vi "am_write_subvi.vi"(6 "Data to Write":u8 format="%.0x", 8 "error in (no error)":errorcluster, 9 "Memory ADD":u16=80 max=1023 format="%.0x", 10 "Aardvark Handle in":i32 min=0, 11 "Address (0x50) in":u16=80 max=1023 format="%.0x") -> (0 "error out":errorcluster, 2 "Dup Aardvark Handle":i32, 3 "Data Written":bool)   [LabVIEW 2014]
uses:
  aardvark.dll
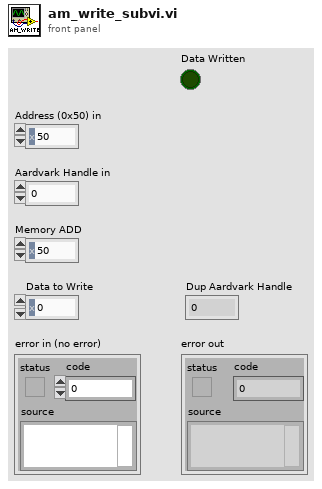
[diagram p1: front panel]
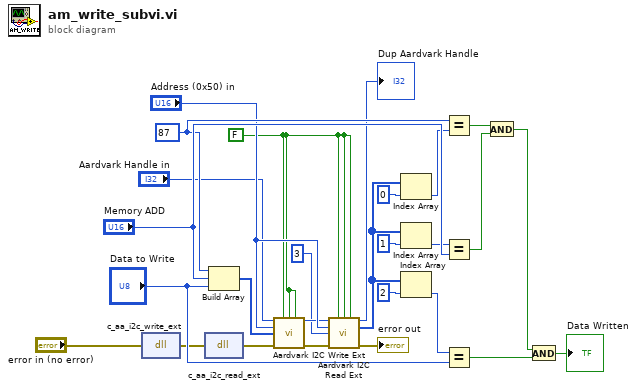
[diagram p0: block diagram]
diagram:
  w8 = FALSE
  w14 = u16 87
  n1 = dll-call lib="aardvark.dll" fn="c_aa_i2c_write_ext"(error in="error in (no error)") -> (error out=w4:errorcluster)  [unwired: 3 in, 1 out]
  n2 = dll-call lib="aardvark.dll" fn="c_aa_i2c_read_ext"(error in=w4) -> (error out=w7:errorcluster)  [unwired: 3 in, 1 out]
  n3 = Build Array(w14, "Memory ADD", "Data to Write") -> (w6:u16[])
  n4 = call <instrlib>:"Aardvark I2C Write Ext.vi"("Aardvark Handle"="Aardvark Handle in", "10-bit Addressing? (False)"=w8, "Combined Format? (False)"=w8, "No Stop? (False)"=w8, "Address (0x50)"="Address (0x50) in", "Data to Write"=w6, "error in (no error)"=w7) -> ("dup Aardvark Handle"=w9:i32, "error out"=w11:errorcluster)  [unwired: 5 in, 2 out]
  n5 = call <instrlib>:"Aardvark I2C Read Ext.vi"("Aardvark Handle"=w9, "10-bit Addressing? (False)"=w8, "Combined Format? (False)"=w8, "No Stop? (False)"=w8, "Address (0x50)"="Address (0x50) in", "Num Bytes to Fetch (64)"=u8 3, "error in (no error)"=w11) -> ("dup Aardvark Handle"=→"Dup Aardvark Handle":i32, "Incoming Data"=w20:u8[], "error out"=→"error out":errorcluster)  [unwired: 5 in, 1 out]
  n6 = Index Array(array=w20, index=0) -> (element=w13:u8)
  n7 = Index Array(array=w20, index=1) -> (element=w17:u8)
  n8 = Index Array(array=w20, index=2) -> (element=w23:u8)
  n9 = Equal?(x=w14, y=w13) -> (x = y?=w18:bool)
  n10 = Equal?(x=w17, y="Memory ADD") -> (x = y?=w19:bool)
  n11 = Equal?(x=w23, y="Data to Write") -> (x = y?=w26:bool)
  n12 = And(x=w18, y=w19) -> (x .and. y?=w22:bool)
  n13 = And(x=w22, y=w26) -> (x .and. y?=→"Data Written":bool)
